vi "Shared Variable Client - Data Item Binding.vi"() -> ()   [LabVIEW 2016]
doc: "This client VI connects to Shared Variable Server.vi by using two of its own shared variables (\"Bound Monitor Value 1\" and \"Bound Monitor Value 2\") that are statically bound to the server's shared variables (\"Monitor Value 1\" and \"Monitor Value 2\")."
panel:
  out "Monitor Value 2":dbl(knob) scale=0.0..1.0
  out "Monitor Value 1":dbl(knob) scale=0.0..1.0
  in  "Stop":bool
  # "Overview: Demonstrates the use of Bound Shared Variables to read shared variable data from a server VI.\nRequirements: Windows\nInstructions:\n1. Make sure Shared Variable Server.vi is already running.\n2. Run this VI. It will read the values of its own shared variables, which are statically bound to the server's shared variables.\n3. Click Stop to stop the VI."
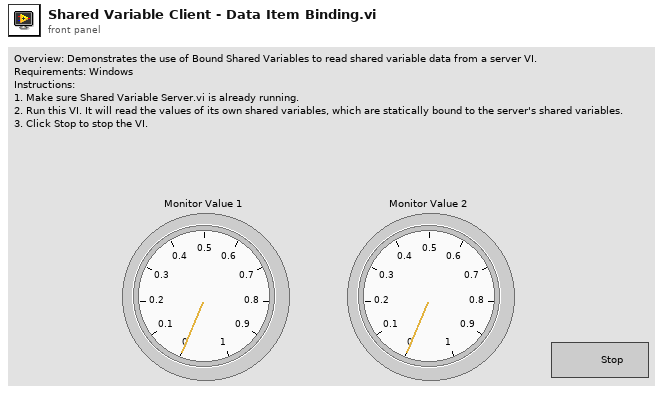
[diagram p1: front panel]
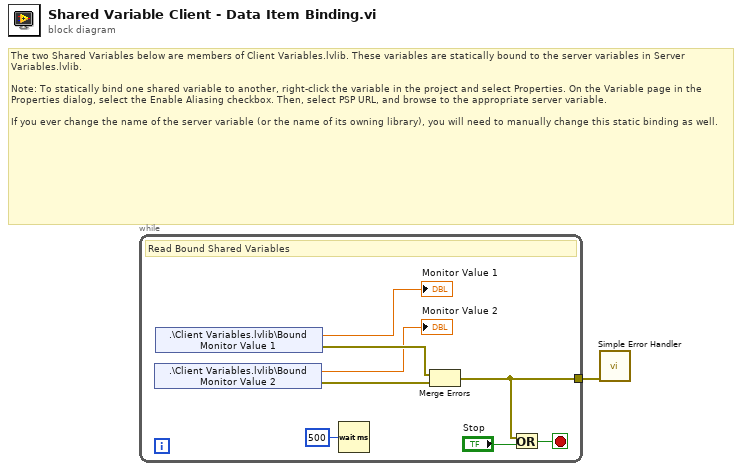
[diagram p0: block diagram]
diagram:
  # "The two Shared Variables below are members of Client Variables.lvlib. These variables are statically bound to the server variables in Server Variables.lvlib.\n\nNote: To statically bind one shared variable to another, right-click the variable in the project and select Properties. On the Variable page in the Properties dialog, select the Enable Aliasing checkbox. Then, select PSP URL, and browse to the appropriate server variable.\n\nIf you ever change the name of the server variable (or the name of its owning library), you will need to manually change this static binding as well."
  n1 = while {
    tunnel: [w4] -> w1
    stop <- w8 stop-if-true
    # "Read Bound Shared Variables"
    n2 = shared-variable ".\\Client Variables.lvlib\\Bound Monitor Value 2"() -> (→"Monitor Value 2":dbl, error out=w6:errorcluster)  [unwired: 1 in]
    n3 = shared-variable ".\\Client Variables.lvlib\\Bound Monitor Value 1"() -> (→"Monitor Value 1":dbl, error out=w5:errorcluster)  [unwired: 1 in]
    n4 = Wait (ms)(milliseconds to wait=u32 500 ("millisecond multiple")) -> ()  [unwired: 1 out]
    n5 = Merge Errors(w5, w6) -> (w4:errorcluster)
    n6 = Or(x=w4, y="Stop") -> (x .or. y?=w8:bool)
  }
  n7 = call <vilib>:"Simple Error Handler.vi"("error in (no error)"=w1) -> ()  [unwired: 4 in, 5 out]
